vi "System Explorer - Copy Templates for System Explorer.vi"(7 "CD Name":string, 8 "error in (no error)":errorcluster, 11 "System Explorer folder":path) -> (0 "error out":errorcluster)   [LabVIEW 2015]
doc: "Copy the templates for the System Explorer library into the System Explorer folder and disconnect the templates from the owning library."
uses:
  Constants/Constants TypDef/CD System Explorer lvlib.ctl
  Constants/Constants TypDef/Common.ctl
  Constants/Constants TypDef/CD Shared lvlib.ctl
  Constants/CD System Explorer lvlib.vi
  Constants/Common.vi
  Constants/CD Shared lvlib.vi
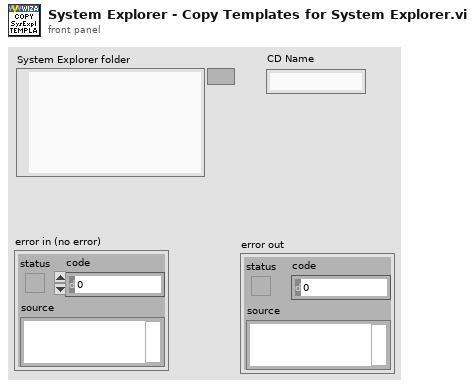
[diagram p1: front panel]
types:
  T1 = typedef "CD System Explorer lvlib.ctl" = enum16{"LibraryFileName", "LibraryFolderName", "System Explorer.FolderName", "System Explorer.Dynamically Called.FolderName", "System Explorer.Dynamically Called.Extra Pages.FolderName", "System Explorer.Dynamically Called.Extra Pages.TemplatePathAndName", "System Explorer.Dynamically Called.Main Page.VIName", "System Explorer.Dynamically Called.Main Page.TemplatePathAndName", "System Explorer.Dynamically Called.Initialization VI.VIName", "System Explorer.Dynamically Called.Initialization VI.TemplatePathAndName", "System Explorer.SubVI.FolderName", "System Explorer.Types.FolderName", "System Explorer.ActionVIOnCompile.VIName", "System Explorer.ExportConfigRTM.VIName"}
  T2 = typedef "CD Shared lvlib.ctl" = enum16{"LibraryFileName", "LibraryFolderName", "ConstantsVI.VIPathAndName", "Shared.FolderName", "Shared.Types.FolderName", "Shared.Constants.VIName", "Shared.Constants.VITemplateName", "Shared.Constants.VITemplatePathAndName", "Shared.CompiledSettings.RelativePath", "Shared.Constants.RelativePath", "Shared.CompiledSettings.Name", "Shared.CompiledSettings.Name.NoExtension", "Shared.CompiledSettings.ClusterName"}
  T3 = typedef "Common.ctl" = enum16{"ProjectName", "TemplatesFolderName", "ProjectTemplatePathAndName", "ReadmeTemplatePathAndName", "TimingAndSyncFolderName", "CustomDeviceFolderName", "PathToTemplates"}
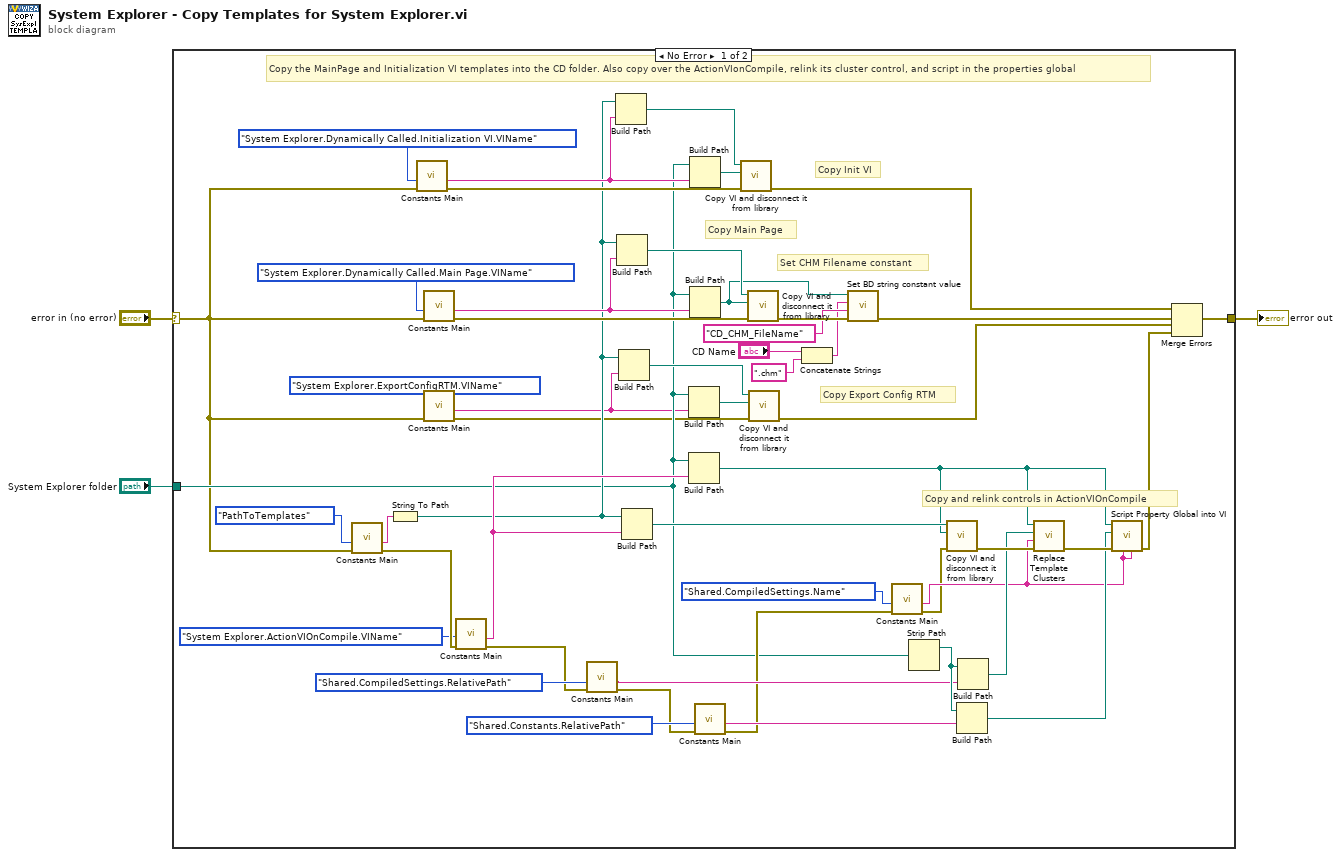
[diagram p0: block diagram]
diagram:
  n1 = case shown="No Error" "error in (no error)" {
    selector: "error in (no error)" -> [w13 w54]
    tunnel: "System Explorer folder" -> [w18 _]
    tunnel: [w47 w54] -> w1
    frame No Error {
      # "Set CHM Filename constant"
      # "Copy Export Config RTM"
      # "Copy and relink controls in ActionVIOnCompile"
      # "Copy Main Page"
      # "Copy Init VI"
      # "Copy the MainPage and Initialization VI templates into the CD folder. Also copy over the ActionVIonCompile, relink its cluster control, and script in the properties global"
      n2 = call-poly "Constants Main.vi"("error in (no error)"=w13, "Action"=Common."PathToTemplates") -> ("error out"=w33:errorcluster, "Output"=w45:string)  [unwired: 8 in]
      n3 = String To Path(string=w45) -> (path=w20:path)
      n4 = call-poly "Constants Main.vi"("error in (no error)"=w13, "Action"=CD_System_Explorer_lvlib."System Explorer.Dynamically Called.Initialization VI.VIName") -> ("error out"=w50:errorcluster, "Output"=w40:string)  [unwired: 8 in]
      n5 = call-poly "Constants Main.vi"("error in (no error)"=w13, "Action"=CD_System_Explorer_lvlib."System Explorer.Dynamically Called.Main Page.VIName") -> ("error out"=w53:errorcluster, "Output"=w39:string)  [unwired: 8 in]
      n6 = call-poly "Constants Main.vi"("error in (no error)"=w13, "Action"=CD_System_Explorer_lvlib."System Explorer.ExportConfigRTM.VIName") -> ("error out"=w16:errorcluster, "Output"=w14:string)  [unwired: 8 in]
      n7 = call-poly "Constants Main.vi"("error in (no error)"=w33, "Action"=CD_System_Explorer_lvlib."System Explorer.ActionVIOnCompile.VIName") -> ("error out"=w26:errorcluster, "Output"=w31:string)  [unwired: 8 in]
      n8 = call-poly "Constants Main.vi"("error in (no error)"=w26, "Action"=CD_Shared_lvlib."Shared.CompiledSettings.RelativePath") -> ("error out"=w25:errorcluster, "Output"=w29:string)  [unwired: 8 in]
      n9 = Build Path(base path=w20, name or relative path=w40) -> (appended path=w41:path)
      n10 = Build Path(base path=w20, name or relative path=w39) -> (appended path=w42:path)
      n11 = Build Path(base path=w20, name or relative path=w14) -> (appended path=w19:path)
      n12 = Build Path(base path=w20, name or relative path=w31) -> (appended path=w44:path)
      n13 = Build Path(base path=w18, name or relative path=w14) -> (appended path=w17:path)
      n14 = Build Path(base path=w18, name or relative path=w31) -> (appended path=w37:path)
      n15 = Build Path(base path=w18, name or relative path=w40) -> (appended path=w49:path)
      n16 = Build Path(base path=w18, name or relative path=w39) -> (appended path=w9:path)
      n17 = call-poly "Constants Main.vi"("error in (no error)"=w25, "Action"=CD_Shared_lvlib."Shared.Constants.RelativePath") -> ("error out"=w22:errorcluster, "Output"=w27:string)  [unwired: 8 in]
      n18 = call "Copy VI and disconnect it from library.vi"("error in (no error)"=w50, "VI Target Path"=w49, "VI Source Path"=w41) -> ("error out"=w48:errorcluster)  [unwired: 8 in]
      n19 = call "Copy VI and disconnect it from library.vi"("error in (no error)"=w53, "VI Target Path"=w9, "VI Source Path"=w42) -> ("error out"=w10:errorcluster)  [unwired: 8 in]
      n20 = call "Copy VI and disconnect it from library.vi"("error in (no error)"=w16, "VI Target Path"=w17, "VI Source Path"=w19) -> ("error out"=w11:errorcluster)  [unwired: 8 in]
      n21 = Concatenate Strings("CD Name", ".chm" ("string")) -> (w5:string)
      n22 = call "Set BD string constant value.vi"("error in (no error)"=w10, "Name of string constant"="CD_CHM_FileName", "New String Value"=w5, "Path to VI"=w9) -> ("error out"=w7:errorcluster)  [unwired: 7 in]
      n23 = call-poly "Constants Main.vi"("error in (no error)"=w22, "Action"=CD_Shared_lvlib."Shared.CompiledSettings.Name") -> ("error out"=w21:errorcluster, "Output"=w24:string)  [unwired: 8 in]
      n24 = Strip Path(path=w18) -> (stripped path=w35:path)  [unwired: 1 out]
      n25 = call "Copy VI and disconnect it from library.vi"("error in (no error)"=w21, "VI Target Path"=w37, "VI Source Path"=w44) -> ("error out"=w43:errorcluster)  [unwired: 8 in]
      n26 = Build Path(base path=w35, name or relative path=w27) -> (appended path=w34:path)
      n27 = Build Path(base path=w35, name or relative path=w29) -> (appended path=w36:path)
      n28 = call "Replace Template Clusters.vi"("error in (no error)"=w43, "Control Name"=w24, "Path to Cluster to Replace"=w36, "Path to VI"=w37) -> ("error out"=w38:errorcluster)  [unwired: 7 in]
      n29 = call "Script Property Global into VI.vi"("GlobalControlName"=w24, "StringConstantToReplace"=w24, "error in (no error)"=w38, "Path to Global"=w34, "Path to VI"=w37) -> ("error out"=w12:errorcluster)  [unwired: 6 in]
      n30 = Merge Errors(w48, w7, w11, w12) -> (w47:errorcluster)
    }
    frame Error {
    }
  }
  "error out" <- w1
